vi "L or R.vi"   [LabVIEW 2020]
uses:
  Variable BX.vi
  RX.vi
  LX.vi
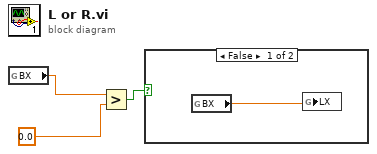
[diagram p0: block diagram]
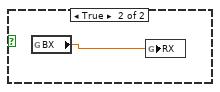
[diagram p2: hidden frame]
diagram:
  n1 = global read "Variable BX.vi" "BX"() -> (w3:dbl)
  n2 = Greater?(x=w3, y=0.0 ("x")) -> (0:w1:bool)
  n3 = case shown="False" w1 {
    frame False {
      n4 = global read "Variable BX.vi" "BX"() -> (w4:dbl)
      n5 = global write "LX.vi" "LX"(w4) -> ()
    }
    frame True {
      n6 = global read "Variable BX.vi" "BX"() -> (w5:dbl)
      n7 = global write "RX.vi" "RX"(w5) -> ()
    }
  }
